vi "Stitching-Generate canvas.vi"(10 "File increment number / Z-plane number":i32, 11 "Canvas template":T1) -> (3 "Stitched image":T1)   [LabVIEW 2013]
uses:
  <vilib>/vision/Image Controls.llb/IMAQ Image.ctl
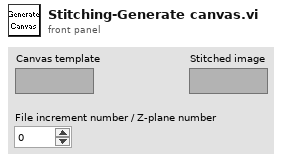
[diagram p1: front panel]
types:
  T1 = typedef "IMAQ Image.ctl" = refnum<image>
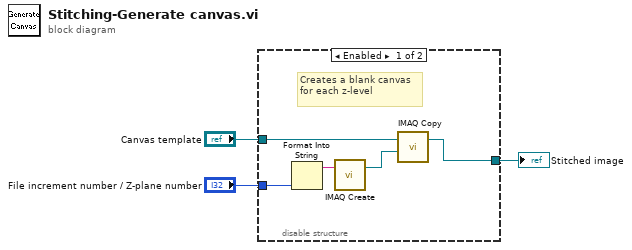
[diagram p0: block diagram]
diagram:
  n1 = disable-structure shown="Enabled" {
    disable-tunnel: [w8 w9] -> w3
    disable-tunnel: "Canvas template" -> [w6 w9]
    disable-tunnel: "File increment number / Z-plane number" -> [w4 _]
    frame Enabled {
      # "Creates a blank canvas for each z-level"
      n2 = Format Into String(w4) -> (resulting string=w5:string)  [unwired: 3 in, 1 out]
      n3 = call "IMAQ Create"("Image Name"=w5) -> ("New Image"=w7:T1)  [unwired: 4 in, 1 out]
      n4 = call "IMAQ Copy"("Image Dst"=w7, "Image Src"=w6) -> ("Image Dst Out"=w8:T1)  [unwired: 4 in, 1 out]
    }
    frame Disabled {
    }
  }
  "Stitched image" <- w3
